vi "Clear.vi"(8 "error in (no error)":errorcluster, 11 "Text Log in":refnum<class "Text Log.lvclass">) -> (0 "error out":errorcluster, 2 "Error Log File Path":path, 3 "Text Log out":refnum<class "Text Log.lvclass">)   [LabVIEW 2020, in "Error Log Classes.lvlib" / "Text Log.lvclass"]
uses:
  Text Log.lvclass
  Text Log.lvclass/Text Log.ctl
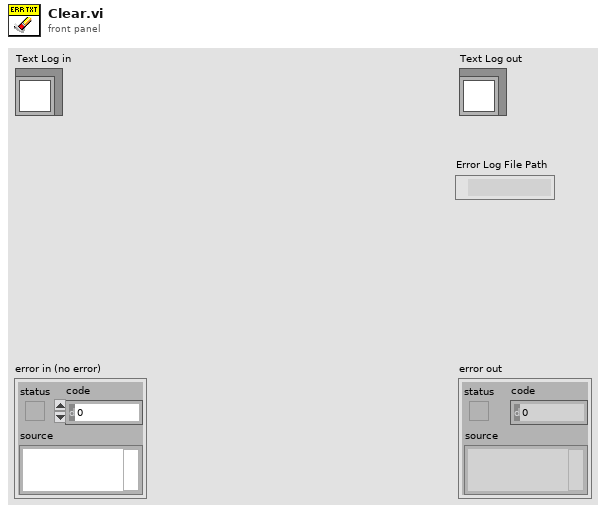
[diagram p1: front panel]
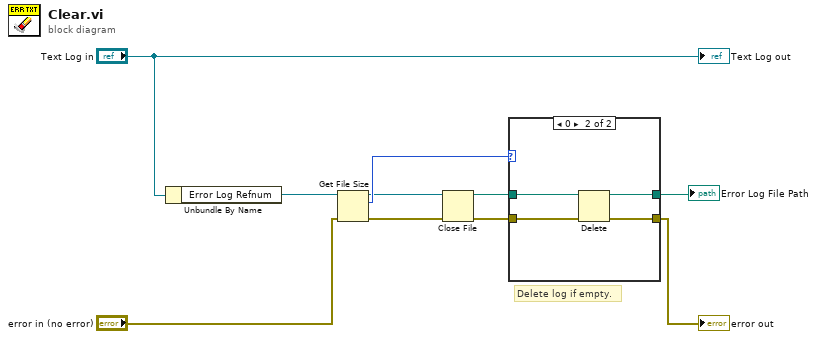
[diagram p0: block diagram]
diagram:
  # "Delete log if empty."
  n1 = Unbundle By Name("Text Log in") -> ("Error Log Refnum"=w4:refnum<file>)
  n2 = Get File Size(file=w4, error in="error in (no error)") -> (refnum out=w7:refnum<file>, size (in bytes)=w9:i64, 0:w6:errorcluster)
  n3 = Close File(refnum=w7, error in=w6) -> (path=w8:path, error out=w10:errorcluster)
  n4 = case shown="0" w9 {
    tunnel: w10 -> [w12 w16]
    tunnel: [w12 w15] -> w2
    tunnel: w8 -> [w11 w14]
    tunnel: [w11 w13] -> w1
    frame Default {
    }
    frame 0 {
      n5 = Delete(path (use dialog)=w14, error in=w16) -> (deleted path=w13:path, error out=w15:errorcluster)  [unwired: 3 in, 1 out]
    }
  }
  "error out" <- w2
  "Error Log File Path" <- w1
  "Text Log out" <- "Text Log in"
